vi "SequenceBuildFromUI.vi"(9 "Attenuations, dB":dbl[](array[numeric]), 10 "Phase Shifts, deg":dbl[](array[numeric]), 11 "2D Selector":bool[][](array[boolean])=[[TRUE, FALSE, FALSE, FALSE, FALSE, FALSE, FALSE, FALSE], [FALSE, FALSE, FALSE, FALSE, FALSE, FALSE, FALSE, FALSE], [TRUE, FALSE, FALSE, FALSE, FALSE, FALSE, FALSE, FALSE], [FALSE, FALSE, FALSE, FALSE, FALSE, FALSE, FALSE, FALSE]] caption="0     1     2     3     4    5     6     7") -> (3 "Test Sequence":T1[](array[typedef]))   [LabVIEW 2017]
uses:
  Classes/Sequence/SequenceSubvis/TestStep.ctl
  Classes/Sequence/SequenceSubvis/RF Direction.ctl
  Classes/Sequence/SequenceSubvis/PolarizationSelect.ctl
panel:
  # "Module #"
  # "Tx"
  # "Rx"
  # "Vertical"
  # "Horizontal"
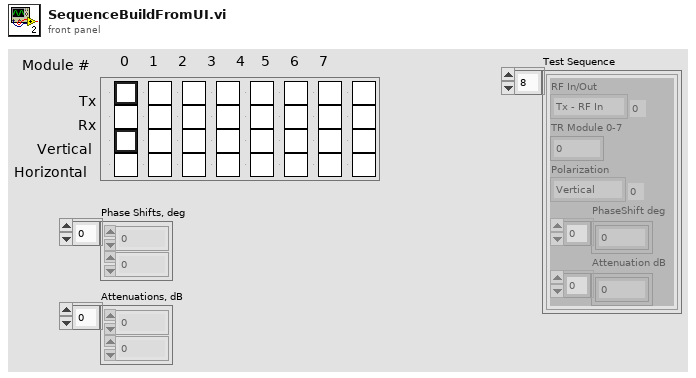
[diagram p1: front panel]
types:
  T1 = typedef "TestStep.ctl" = cluster{"RF In/Out":T2, "TR Module 0-7":i32, "Polarization":T3, "PhaseShift deg":dbl[], "Attenuation dB":dbl[]}
  T2 = typedef "RF Direction.ctl" = enum16{"Tx - RF In", "Rx - RF Out"}
  T3 = typedef "PolarizationSelect.ctl" = enum16{"Vertical", "Horizontal"}
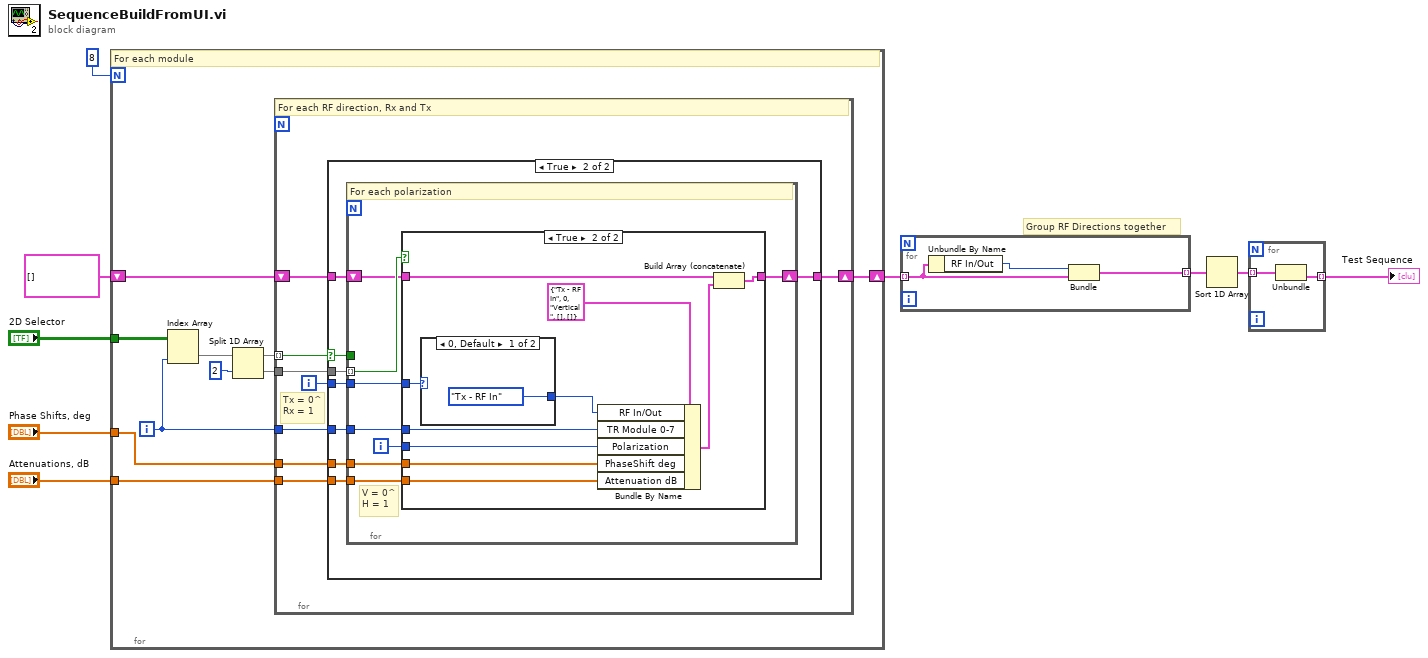
[diagram p0: block diagram]
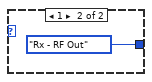
[diagram p4: hidden frame]
diagram:
  # "Group RF Directions together"
  n1 = for {
    N: 8 -> [_]
    tunnel: "2D Selector" -> [w19]
    shift-right: [w11] -> w4
    shift-left: T1[] [] -> [w15]
    tunnel: "Phase Shifts, deg" -> [w13]
    tunnel: "Attenuations, dB" -> [w12]
    i -> [w14]
    # "For each module"
    n2 = Index Array(array=w19, index (col)=w14) -> (element=w18:bool[])  [unwired: 1 in]
    n3 = Split 1D Array(array=w18, index=2) -> (first subarray=w17:bool[], second subarray=w16:bool[])
    n4 = for {
      tunnel: w17 -> [w26] mode=indexing
      tunnel: w16 -> [w27]
      shift-right: [w20] -> w11
      shift-left: w15 -> [w25]
      tunnel: w14 -> [w23]
      tunnel: w13 -> [w22]
      tunnel: w12 -> [w21]
      i -> [w24]
      # "Tx = 0^\nRx = 1"
      # "For each RF direction, Rx and Tx"
      n5 = case shown="True" w26 {
        selector: w26 -> [_ w35]
        tunnel: w27 -> [_ w36]
        tunnel: w25 -> [w28 w34]
        tunnel: w24 -> [_ w33]
        tunnel: w23 -> [_ w32]
        tunnel: w22 -> [_ w31]
        tunnel: w21 -> [_ w30]
        tunnel: [w28 w29] -> w20
        frame False {
        }
        frame True {
          n6 = for {
            tunnel: w36 -> [w44] mode=indexing
            tunnel: w35 -> [_]
            shift-right: [w38] -> w29
            shift-left: w34 -> [w37]
            tunnel: w33 -> [w43]
            tunnel: w32 -> [w42]
            tunnel: w31 -> [w40]
            tunnel: w30 -> [w39]
            i -> [w41]
            # "V = 0^\nH = 1"
            # "For each polarization"
            n7 = case shown="True" w44 {
              tunnel: w43 -> [_ w55]
              tunnel: w42 -> [_ w52]
              tunnel: w41 -> [_ w51]
              tunnel: w40 -> [_ w50]
              tunnel: w39 -> [_ w49]
              tunnel: [w45 w47] -> w38
              tunnel: w37 -> [w45 w46]
              frame False {
              }
              frame True {
                n8 = case shown="0, Default" w55 {
                  tunnel: [RF_Direction."Tx - RF In" ("RF In/Out") RF_Direction."Rx - RF Out" ("RF In/Out")] -> w53
                  frame 0, Default {
                  }
                  frame 1 {
                  }
                }
                n9 = Bundle By Name(cluster=T1 {"RF In/Out"=enum."Tx - RF In", "TR Module 0-7"=0, "Polarization"=enum."Vertical", "PhaseShift deg"=[], "Attenuation dB"=[]} ("Test"), "RF In/Out"=w53, "TR Module 0-7"=w52, "Polarization"=w51, "PhaseShift deg"=w50, "Attenuation dB"=w49) -> (w48:T1)
                n10 = Build Array (concatenate)(w46, w48) -> (w47:T1[])
              }
            }
          }
        }
      }
    }
  }
  n11 = for {
    tunnel: w4 -> [w59] mode=indexing
    tunnel: [w58] -> w3 mode=indexing
    n12 = Unbundle By Name(w59) -> ("RF In/Out"=w60:T2)
    n13 = Bundle("RF In/Out"=w60, "Test"=w59) -> (w58:cluster{"RF In/Out":T2, "Test":T1})  [unwired: 1 in]
  }
  n14 = Sort 1D Array(array=w3) -> (sorted array=w2:cluster{"RF In/Out":T2, "Test":T1}[])
  n15 = for {
    tunnel: w2 -> [w62] mode=indexing
    tunnel: [w61] -> w1 mode=indexing
    n16 = Unbundle(w62) -> ("Test"=w61:T1)  [unwired: 1 out]
  }
  "Test Sequence" <- w1
